vi "Precheck.vi"(6 "Using Lamps":bool, 7 "Current Lamp cluster":T1, 9 "Target info":cluster{"RA":string, "DEC":string}, 10 "cluster":T2={"SI camera info"={"Observer Name"="", "object name"="", "File name base"="", "Camera Color"="Red", "Exp type tab"="", "Number of Exp"=1, "Exp time"=0, "CCD Readout Speed"=5, "CCD ROI Mode"=10, "Hg(Ar)"=FALSE, "Cu"=FALSE, "Ne"=FALSE, "Bulb"=FALSE, "Ar"=FALSE, "Quartz"=FALSE, "Quartz Percent"=0, "Fe"=FALSE, "Notes"="", "Target Number"="", "DomePercent"=0, "Dome"=FALSE, "Start"=0.0, "Delta"=0.0, "Steps"=0.0, "Custom Roi"={0, 4096, 1, 0, 4096, 1}}, "Configuration"={"Primary Filter"="<NO FILTER>", "Secondary Filter"="<NO FILTER>", "Slit Mask"="<NO MASK>", "Grating"="<NO GRATING>", "CS Target"=0.0, "GS Target"=0.0, "Coll Focus"=1000, "Camera Focus"=0, "Name"="", "User"="", "Date"="", "Comment"="", "use Flexure Comp?"=TRUE, "Select Mode:"=0}, "RA (HH:MM:SS.SS)"="-00:00:00.00", "DEC (HH:MM:SS.SS)"="-00:00:00.00"} {"Configuration"."Select Mode:" items=["Custom", "Imaging", "300 All", "600 UV", "600 Blue", "600 Mid", "600 Red", "1200 m0", "1200 m1", "1200 m2", "1200 m3", "1200 m4", "1200 m5", "1200 m6", "1200 m7", "1200 RESOLVE", "400 m1", "400 m2", "930 m1", "930 m2", "930 m3", "930 m4", "930 m5", "930 m6", "400WD", "930TP", "400Fermi", "400Padgett", "400Lewis", "400Crotts", "600BLee", "600RLee", "400WW"]; "SI camera info"."DomePercent" min=0 step=1; "SI camera info"."Quartz Percent" min=0 step=1; "SI camera info"."CCD Readout Speed" items=["750 kHz, ATTN 0", "750 kHz, ATTN 2", "344 kHz, ATTN 0", "344 kHz, ATTN 3", "100 kHz, ATTN 2", "100 kHz, ATTN 3"]; "SI camera info"."CCD ROI Mode" items=["Imaging, 1x1  "=0, "Imaging, 2x2"=1, "Imaging, 3x3"=2, "Spectroscopic, 1x1"=3, "Spectroscopic, 2x2"=4, "Spectroscopic, 3x3"=5, "MOS, 1x1"=11, "MOS, 2x2"=12, "MOS, 3x3"=13, "Slicer"=6, "Spectroscopic, ZZ Ceti"=14, "Slit Imaging/Alignment"=7, "MOS Imaging/Alignment"=10, "Set user-defined ROI..."=21, "Custom Mode"=9]; "SI camera info"."Number of Exp" min=0 step=1; "SI camera info"."Exp time" min=0 step=1}, 11 "line number":dbl) -> (1 "Comp Mirror in?":bool, 2 "Lamp Pause":bool, 3 "Target Pause":bool, 4 "Change Lamps":bool, 5 "Using Lamps Out":bool)   [LabVIEW 2015]
uses:
  Users/Sherman/Desktop/BETA_GSCS/Systems/TCS_Link/TCSLINK_global.vi
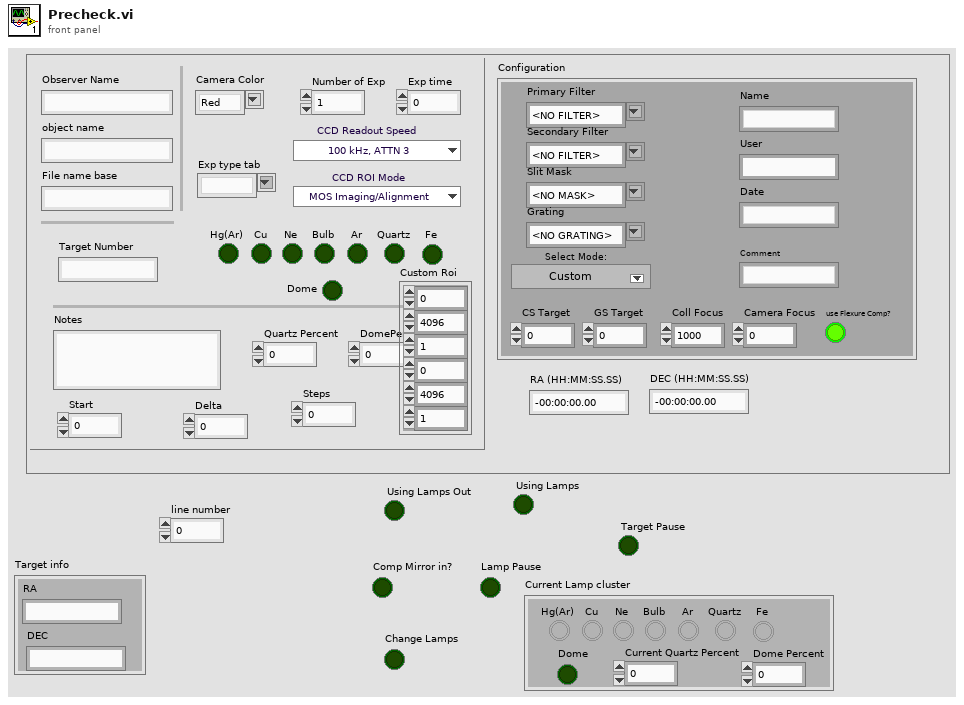
[diagram p1: front panel]
types:
  T1 = cluster{"Bulb":bool, "Fe":bool, "Quartz":bool, "Ar":bool, "Ne":bool, "Cu":bool, "Hg(Ar)":bool, "Current Quartz Percent":dbl, "Dome":bool, "Dome Percent":dbl}
  T2 = cluster{"SI camera info":cluster{"Observer Name":string, "object name":string, "File name base":string, "Camera Color":string, "Exp type tab":string, "Number of Exp":i32, "Exp time":i32, "CCD Readout Speed":u8, "CCD ROI Mode":u16, "Hg(Ar)":bool, "Cu":bool, "Ne":bool, "Bulb":bool, "Ar":bool, "Quartz":bool, "Quartz Percent":i32, "Fe":bool, "Notes":string, "Target Number":string, "DomePercent":i32, "Dome":bool, "Start":dbl, "Delta":dbl, "Steps":dbl, "Custom Roi":cluster{i32, i32, i32, i32, i32, i32}}, "Configuration":cluster{"Primary Filter":string, "Secondary Filter":string, "Slit Mask":string, "Grating":string, "CS Target":dbl, "GS Target":dbl, "Coll Focus":i32, "Camera Focus":i32, "Name":string, "User":string, "Date":string, "Comment":string, "use Flexure Comp?":bool, "Select Mode:":u16}, "RA (HH:MM:SS.SS)":string, "DEC (HH:MM:SS.SS)":string}
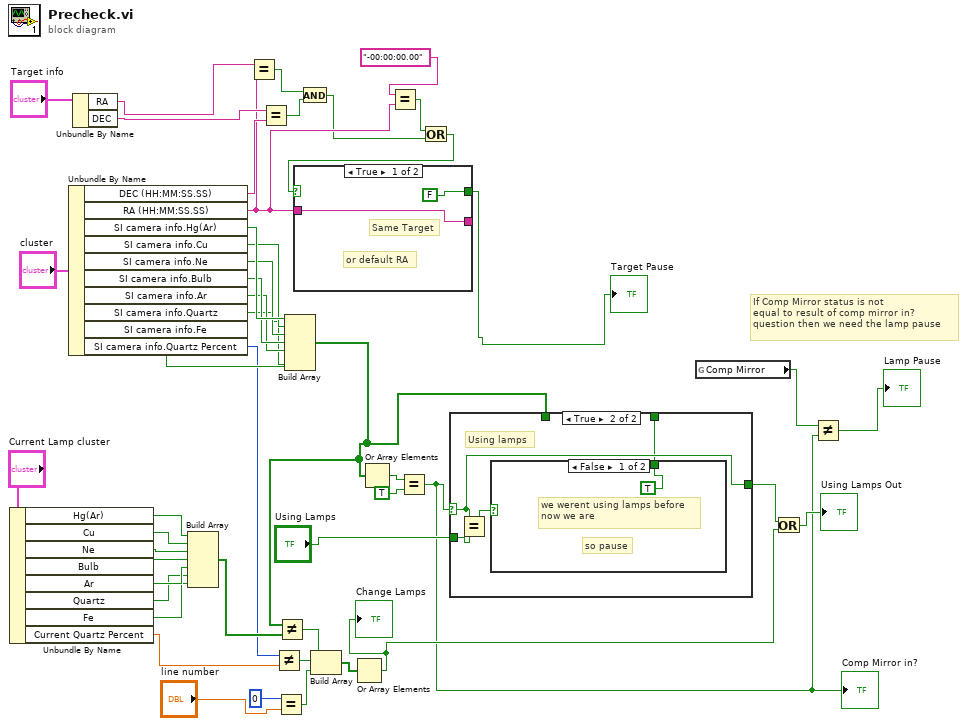
[diagram p0: block diagram]
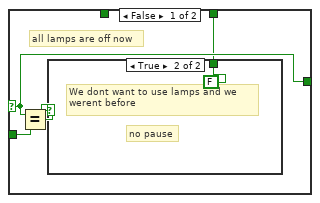
[diagram p2: hidden frame]
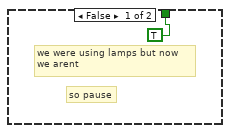
[diagram p3: hidden frame]
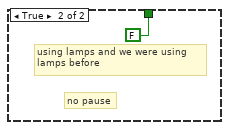
[diagram p4: hidden frame]
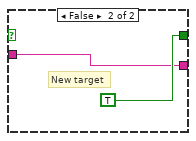
[diagram p5: hidden frame]
diagram:
  # "If Comp Mirror status is not \nequal to result of comp mirror in? \nquestion then we need the lamp pause"
  n1 = Unbundle By Name("Current Lamp cluster") -> ("Hg(Ar)"=w34:bool, "Cu"=w33:bool, "Ne"=w32:bool, "Bulb"=w31:bool, "Ar"=w30:bool, "Quartz"=w29:bool, "Fe"=w28:bool, "Current Quartz Percent"=w24:dbl)
  n2 = Unbundle By Name("cluster") -> ("DEC (HH:MM:SS.SS)"=w10:string, "RA (HH:MM:SS.SS)"=w4:string, "SI camera info.Hg(Ar)"=w46:bool, "SI camera info.Cu"=w45:bool, "SI camera info.Ne"=w44:bool, "SI camera info.Bulb"=w43:bool, "SI camera info.Ar"=w42:bool, "SI camera info.Quartz"=w41:bool, "SI camera info.Fe"=w40:bool, "SI camera info.Quartz Percent"=w25:i32)
  n3 = Unbundle By Name("Target info") -> ("RA"=w9:string, "DEC"=w8:string)
  n4 = Build Array(w34, w33, w32, w31, w30, w29, w28) -> (w26:bool[])
  n5 = Equal?(x=w9, y=w4) -> (x = y?=w7:bool)
  n6 = Equal?(x=w8, y=w10) -> (x = y?=w6:bool)
  n7 = Not Equal?(x=w25, y=w24) -> (x != y?=w20:bool)
  n8 = Equal?(x=0, y="line number") -> (x = y?=w19:bool)
  n9 = Build Array(w46, w45, w44, w43, w42, w41, w40) -> (w27:bool[])
  n10 = Not Equal?(x=w27, y=w26) -> (x != y?=w21:bool)
  n11 = And(x=w7, y=w6) -> (x .and. y?=w3:bool)
  n12 = Build Array(w21, w20, w19) -> (w18:bool[])
  n13 = Or Array Elements(Boolean array=w18) -> (logical OR=w15:bool)
  "Change Lamps" <- w15
  n14 = Or Array Elements(Boolean array=w27) -> (logical OR=w39:bool)
  n15 = Equal?(x="-00:00:00.00", y=w4) -> (x = y?=w2:bool)
  n16 = Equal?(x=w39, y=TRUE) -> (x = y?=w13:bool)
  "Comp Mirror in?" <- w13
  n17 = Or(x=w2, y=w3) -> (x .or. y?=w1:bool)
  n18 = case shown="True" w1 {
    tunnel: w4 -> [w49 w50]
    tunnel: [FALSE TRUE] -> w36
    tunnel: [w49 w50] -> _
    frame True {
      # "or default RA"
      # "Same Target"
    }
    frame False {
      # "New target"
    }
  }
  "Target Pause" <- w36
  n19 = case shown="True" w13 {
    selector: w13 -> [w54 w59]
    tunnel: [w53 w58] -> _
    tunnel: w27 -> [_ _]
    tunnel: "Using Lamps" -> [w55 w61]
    tunnel: [w54 w59] -> w17
    frame False {
      # "all lamps are off now"
      n20 = Equal?(x=w54, y=w55) -> (x = y?=w52:bool)
      n21 = case shown="True" w52 {
        tunnel: [TRUE FALSE] -> w53
        frame False {
          # "so pause"
          # "we were using lamps but now\nwe arent"
        }
        frame True {
          # "no pause"
          # "We dont want to use lamps and we \nwerent before"
        }
      }
    }
    frame True {
      # "Using lamps"
      n22 = Equal?(x=w59, y=w61) -> (x = y?=w60:bool)
      n23 = case shown="False" w60 {
        tunnel: [TRUE FALSE] -> w58
        frame False {
          # "so pause"
          # "we werent using lamps before\nnow we are"
        }
        frame True {
          # "no pause"
          # "using lamps and we were using \nlamps before"
        }
      }
    }
  }
  n24 = global read "TCSLINK_global.vi" "Comp Mirror"() -> (w14:bool)
  n25 = Or(x=w17, y=w15) -> (x .or. y?=→"Using Lamps Out":bool)
  n26 = Not Equal?(x=w14, y=w13) -> (x != y?=→"Lamp Pause":bool)
